vi "to string.vi"(8 "error in":errorcluster, 11 "SwitchACIR configuration":refnum<class "SwitchACIR Channel configuration.lvclass">) -> (0 "error out":errorcluster, 1 "data":string, 2 "version":string, 3 "SwitchACIR configuration out":refnum<class "SwitchACIR Channel configuration.lvclass">)   [LabVIEW 2025, in "SwitchACIR Channel configuration.lvclass"]
doc: "Provides an interface for saving a module configuration to a file or other serialized data source. It is recommended that all children of this class store data in two sets--data required for its own initialization, and any data required for parent initialization--and that each implementation uses the <b>Call Parent Method</b> primitive to serialize parent information.Copyright 2017 National Instruments Corporation\n\nLicensed under the Apache License, Version 2.0 (the \"License\"); you may not use this file except in compliance with the License. You may obtain a copy of the License at http://www.apache.org/licenses/LICENSE-2.0\nUnless required by applicable law or agreed to in writing, software distributed under the License is distributed on an \"AS IS\" BASIS, WITHOUT WARRANTIES OR CONDITIONS OF ANY KIND, either express or implied. See the License for the specific language governing permissions and limitations under the License."
uses:
  SwitchACIR Channel configuration.lvclass
  SwitchACIR Channel configuration.lvclass/SwitchACIR Channel configuration.ctl
  Users/Public/Documents/Sandia National Labs/TSS Plugin/Abstract Engine.lvlibp/Plugin/Abstract/Channel configuration/Channel configuration.lvclass
  Users/Public/Documents/Sandia National Labs/TSS Plugin/CEF.lvlibp/serializable configuration/CEF_serializable configuration.lvclass
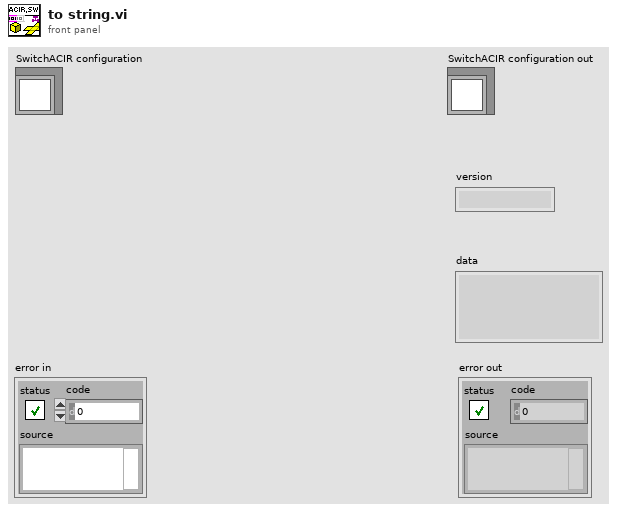
[diagram p1: front panel]
types:
  T1 = typedef "SwitchACIR Channel configuration.lvclass/SwitchACIR Channel Setting.ctl" = cluster{"Switch":string}
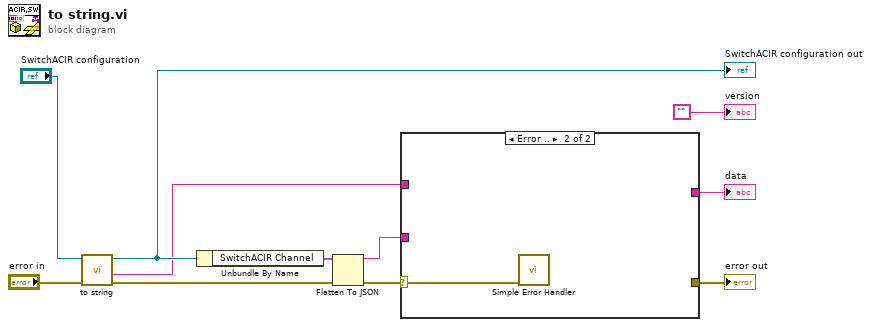
[diagram p0: block diagram]
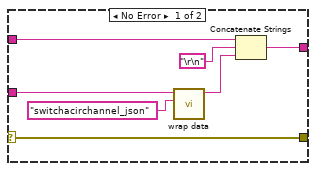
[diagram p2: hidden frame]
diagram:
  n1 = call-parent "to string.vi"("error in"="error in", "Channel configuration"="SwitchACIR configuration") -> ("error out"=w11:errorcluster, "data"=w2:string, "Channel configuration out"=w7:refnum<class "SwitchACIR Channel configuration.lvclass">)  [unwired: 6 in, 1 out]
  "SwitchACIR configuration out" <- w7
  n2 = Unbundle By Name(w7) -> ("SwitchACIR Channel"=w9:T1)
  n3 = Flatten To JSON(anything=w9, error in (no error)=w11) -> (JSON string=w4:string, 11:w6:errorcluster)  [unwired: 1 in]
  n4 = case shown="Error .." w6 {
    selector: w6 -> [w18 w19]
    tunnel: [w18 _] -> w5
    tunnel: w4 -> [w15 _]
    tunnel: w2 -> [w14 _]
    tunnel: [w12 _] -> w3
    frame No Error {
      n5 = call "wrap data.vi"("identifier"="switchacirchannel_json" ("additional identifier"), "data to wrap"=w15) -> ("wrapped data"=w17:string)  [unwired: 9 in]
      n6 = Concatenate Strings(w14, "\r\n", w17) -> (w12:string)
    }
    frame Error {
      n7 = call <vilib>:"Simple Error Handler.vi"("error in (no error)"=w19) -> ()  [unwired: 4 in, 5 out]
    }
  }
  "error out" <- w5
  "data" <- w3
  "version" <- ""
